vi "set_material_parameters_cluster.vi"(8 "error in (no error)":errorcluster, 9 "Material parameters":T1, 10 "Material number":u8, 11 "VISA resource name":refnum<visa-resource-name>) -> (0 "error out":errorcluster, 3 "VISA resource name out":refnum<visa-resource-name>)   [LabVIEW 2018]
doc: "Set the density of a material."
uses:
  Low Level/material_parameter_ring.ctl
  Low Level/material_parameters.ctl
panel:
  out "Label.Text":string
  in  "Material parameter":T2 items=["Density (g/cc)", "Z-Ratio", "Master Tooling (%)", "Control Loop", "Process Gain (A/s/%)", "Time Constant (s)", "Dead Time (s)", "Source", "Maximum Power (%)", "Minimum Power (%)", "Max Power Option", "PreCond Soak Power (%)", "PreCond Rise Time (s) (mm:ss)", "PreCond Soak Time (s) (mm:ss)", "Soak Power 1 (%)", "Rise Time 1 (s) (mm:ss)", "Soak Time 1 (s) (mm:ss)", "Soak Power 2 (%)", "Rise Time 2 (s) (mm:ss)", "Soak Time 2 (s) (mm:ss)", "Auto Soak 2", "Dep After Pre-Dep", "Delay Option", "Control Delay Time (s) (mm:ss)", "Shutter Delay Accur (%)", "Transfer Sensor", "Transfer Tooling (%)", "Feed Power (%)", "Feed Ramp Time (s) (mm:ss)", "Feed Time (s) (mm:ss)", "Idle Power (%)", "Idle Ramp Time (s) (mm:ss)", "Rate (A/s)", "Time Limit (s) (mm:ss)", "Rate Filter Time (s)", "Time Power Avg Time (minutes)", "Ion Assist Deposit", "On Final Thickness", "Ramp 1 Rate (A/s)", "Start Ramp 1 (kA)", "Ramp 1 Time (s) (mm:ss)", "Ramp 2 Rate (A/s)", "Start Ramp 2 (kA)", "Ramp 2 Time (s) (mm:ss)", "RateWatcher Option", "RateWatcher Time (s) (mm:ss)", "RateWatcher Accuracy (%)", "Multipoint", "Aggregate Multiplier", "Sensor 1 Failure Action", "Sensor 2 Failure Action", "Sensor 3 Failure Action", "Sensor 4 Failure Action", "Sensor 5 Failure Action", "Sensor 6 Failure Action", "Sensor 7 Failure Action", "Sensor 8 Failure Action", "Sensor 1 Failure Trigger", "Sensor 2 Failure Trigger", "Sensor 3 Failure Trigger", "Sensor 4 Failure Trigger", "Sensor 5 Failure Trigger", "Sensor 6 Failure Trigger", "Sensor 7 Failure Trigger", "Sensor 8 Failure Trigger", "Sensor 1 Weight (%)", "Sensor 2 Weight (%)", "Sensor 3 Weight (%)", "Sensor 4 Weight (%)", "Sensor 5 Weight (%)", "Sensor 6 Weight (%)", "Sensor 7 Weight (%)", "Sensor 8 Weight (%)", "Sensor 1 Tooling (%)", "Sensor 2 Tooling (%)", "Sensor 3 Tooling (%)", "Sensor 4 Tooling (%)", "Sensor 5 Tooling (%)", "Sensor 6 Tooling (%)", "Sensor 7 Tooling (%)", "Sensor 8 Tooling (%)", "Sensor 1 CrystalTwo Tooling (%)", "Sensor 2 CrystalTwo Tooling (%)", "Sensor 3 CrystalTwo Tooling (%)", "Sensor 4 CrystalTwo Tooling (%)", "Sensor 5 CrystalTwo Tooling (%)", "Sensor 6 CrystalTwo Tooling (%)", "Sensor 7 CrystalTwo Tooling (%)", "Sensor 8 CrystalTwo Tooling (%)", "Sensor 1 Cal Thickness (kA)", "Sensor 2 Cal Thickness (kA)", "Sensor 3 Cal Thickness (kA)", "Sensor 4 Cal Thickness (kA)", "Sensor 5 Cal Thickness (kA)", "Sensor 6 Cal Thickness (kA)", "Sensor 7 Cal Thickness (kA)", "Sensor 8 Cal Thickness (kA)", "Sensor 1 Xtal Position First", "Sensor 2 Xtal Position First", "Sensor 3 Xtal Position First", "Sensor 4 Xtal Position First", "Sensor 5 Xtal Position First", "Sensor 6 Xtal Position First", "Sensor 7 Xtal Position First", "Sensor 8 Xtal Position First", "Sensor 1 Xtal Position Last", "Sensor 2 Xtal Position Last", "Sensor 3 Xtal Position Last", "Sensor 4 Xtal Position Last", "Sensor 5 Xtal Position Last", "Sensor 6 Xtal Position Last", "Sensor 7 Xtal Position Last", "Sensor 8 Xtal Position Last", "Sensor", "Failure Action", "CrystalTwo Tooling (%)", "Xtal Position First", "Xtal Position Last", "Backup Sensor", "Backup Tooling (%)", "Quality Percent (%)", "Quality Counts", "Stability Single (Hz)", "Stability Total (Hz)", "Recorder Output", "Recorder Function", "Recorder Range"]
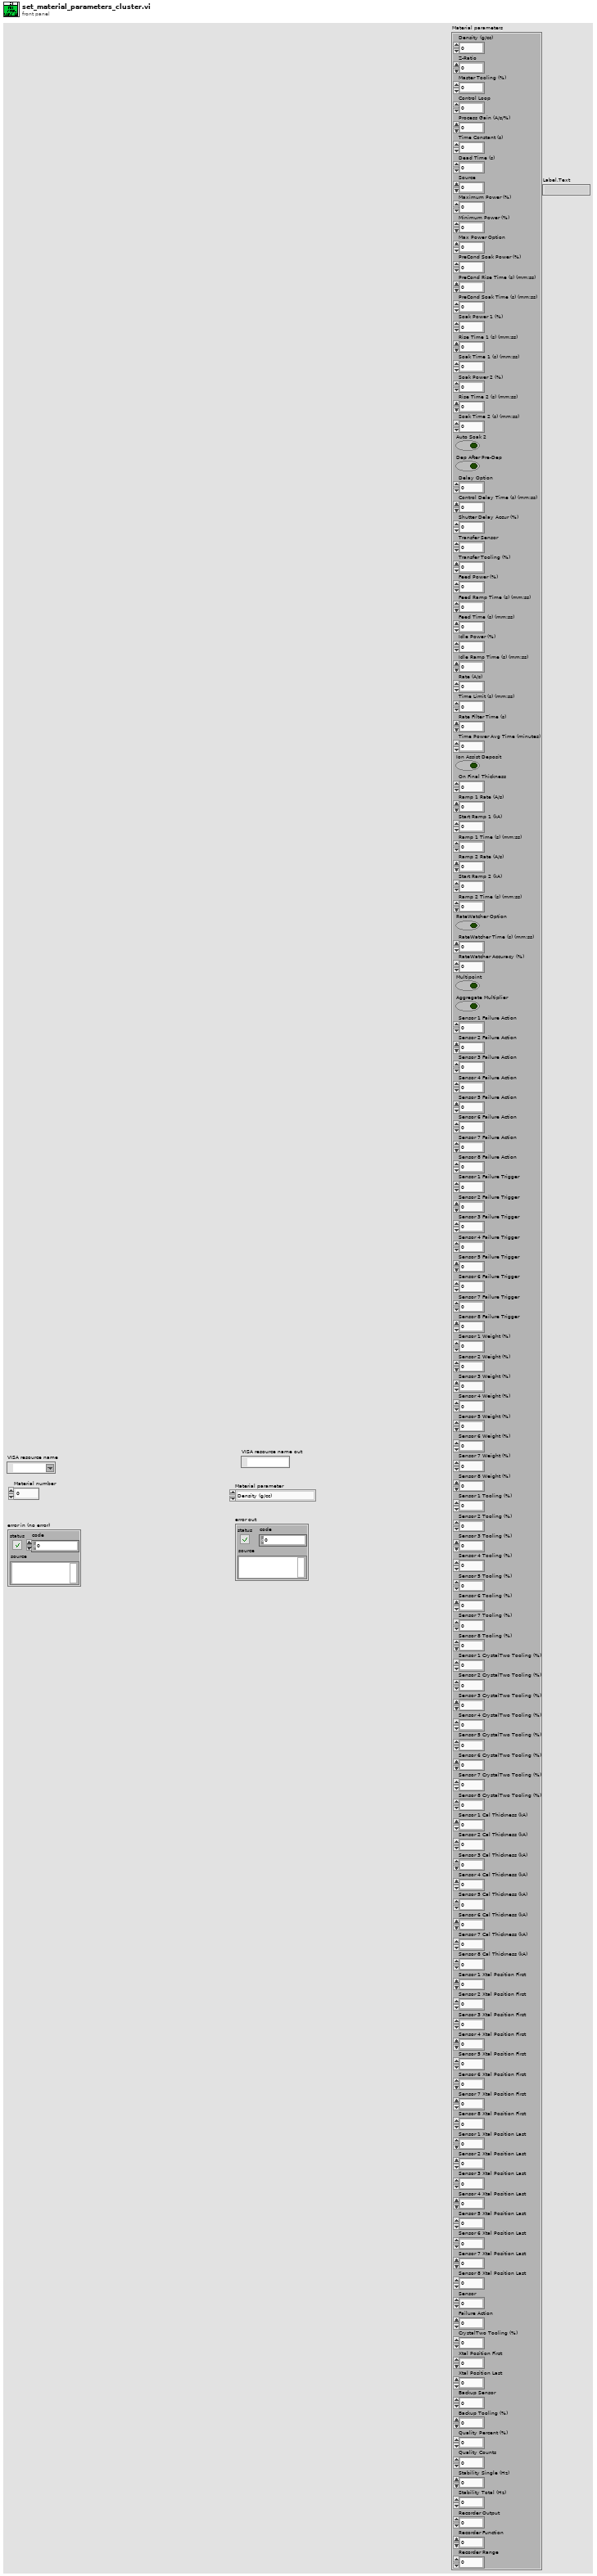
[diagram p1: front panel]
types:
  T1 = typedef "material_parameters.ctl" = cluster{"Density (g/cc)":sgl, "Z-Ratio":sgl, "Master Tooling (%)":sgl, "Control Loop":u8, "Process Gain (A/s/%)":sgl, "Time Constant (s)":sgl, "Dead Time (s)":sgl, "Source":u8, "Maximum Power (%)":sgl, "Minimum Power (%)":sgl, "Max Power Option":u8, "PreCond Soak Power (%)":sgl, "PreCond Rise Time (s) (mm:ss)":u16, "PreCond Soak Time (s) (mm:ss)":u16, "Soak Power 1 (%)":sgl, "Rise Time 1 (s) (mm:ss)":u16, "Soak Time 1 (s) (mm:ss)":u16, "Soak Power 2 (%)":sgl, "Rise Time 2 (s) (mm:ss)":u16, "Soak Time 2 (s) (mm:ss)":u16, "Auto Soak 2":bool, "Dep After Pre-Dep":bool, "Delay Option":u8, "Control Delay Time (s) (mm:ss)":u16, "Shutter Delay Accur (%)":u8, "Transfer Sensor":u8, "Transfer Tooling (%)":sgl, "Feed Power (%)":sgl, "Feed Ramp Time (s) (mm:ss)":u16, "Feed Time (s) (mm:ss)":u16, "Idle Power (%)":sgl, "Idle Ramp Time (s) (mm:ss)":u16, "Rate (A/s)":sgl, "Time Limit (s) (mm:ss)":u16, "Rate Filter Time (s)":u8, "Time Power Avg Time (minutes)":u8, "Ion Assist Deposit":bool, "On Final Thickness":u8, "Ramp 1 Rate (A/s)":sgl, "Start Ramp 1 (kA)":sgl, "Ramp 1 Time (s) (mm:ss)":u16, "Ramp 2 Rate (A/s)":sgl, "Start Ramp 2 (kA)":sgl, "Ramp 2 Time (s) (mm:ss)":u16, "RateWatcher Option":bool, "RateWatcher Time (s) (mm:ss)":u16, "RateWatcher Accuracy (%)":u8, "Multipoint":bool, "Aggregate Multiplier":bool, "Sensor 1 Failure Action":u8, "Sensor 2 Failure Action":u8, "Sensor 3 Failure Action":u8, "Sensor 4 Failure Action":u8, "Sensor 5 Failure Action":u8, "Sensor 6 Failure Action":u8, "Sensor 7 Failure Action":u8, "Sensor 8 Failure Action":u8, "Sensor 1 Failure Trigger":u8, "Sensor 2 Failure Trigger":u8, "Sensor 3 Failure Trigger":u8, "Sensor 4 Failure Trigger":u8, "Sensor 5 Failure Trigger":u8, "Sensor 6 Failure Trigger":u8, "Sensor 7 Failure Trigger":u8, "Sensor 8 Failure Trigger":u8, "Sensor 1 Weight (%)":sgl, "Sensor 2 Weight (%)":sgl, "Sensor 3 Weight (%)":sgl, "Sensor 4 Weight (%)":sgl, "Sensor 5 Weight (%)":sgl, "Sensor 6 Weight (%)":sgl, "Sensor 7 Weight (%)":sgl, "Sensor 8 Weight (%)":sgl, "Sensor 1 Tooling (%)":sgl, "Sensor 2 Tooling (%)":sgl, "Sensor 3 Tooling (%)":sgl, "Sensor 4 Tooling (%)":sgl, "Sensor 5 Tooling (%)":sgl, "Sensor 6 Tooling (%)":sgl, "Sensor 7 Tooling (%)":sgl, "Sensor 8 Tooling (%)":sgl, "Sensor 1 CrystalTwo Tooling (%)":sgl, "Sensor 2 CrystalTwo Tooling (%)":sgl, "Sensor 3 CrystalTwo Tooling (%)":sgl, "Sensor 4 CrystalTwo Tooling (%)":sgl, "Sensor 5 CrystalTwo Tooling (%)":sgl, "Sensor 6 CrystalTwo Tooling (%)":sgl, "Sensor 7 CrystalTwo Tooling (%)":sgl, "Sensor 8 CrystalTwo Tooling (%)":sgl, "Sensor 1 Cal Thickness (kA)":sgl, "Sensor 2 Cal Thickness (kA)":sgl, "Sensor 3 Cal Thickness (kA)":sgl, "Sensor 4 Cal Thickness (kA)":sgl, "Sensor 5 Cal Thickness (kA)":sgl, "Sensor 6 Cal Thickness (kA)":sgl, "Sensor 7 Cal Thickness (kA)":sgl, "Sensor 8 Cal Thickness (kA)":sgl, "Sensor 1 Xtal Position First":u8, "Sensor 2 Xtal Position First":u8, "Sensor 3 Xtal Position First":u8, "Sensor 4 Xtal Position First":u8, "Sensor 5 Xtal Position First":u8, "Sensor 6 Xtal Position First":u8, "Sensor 7 Xtal Position First":u8, "Sensor 8 Xtal Position First":u8, "Sensor 1 Xtal Position Last":u8, "Sensor 2 Xtal Position Last":u8, "Sensor 3 Xtal Position Last":u8, "Sensor 4 Xtal Position Last":u8, "Sensor 5 Xtal Position Last":u8, "Sensor 6 Xtal Position Last":u8, "Sensor 7 Xtal Position Last":u8, "Sensor 8 Xtal Position Last":u8, "Sensor":u8, "Failure Action":u8, "CrystalTwo Tooling (%)":sgl, "Xtal Position First":u8, "Xtal Position Last":u8, "Backup Sensor":u8, "Backup Tooling (%)":sgl, "Quality Percent (%)":u8, "Quality Counts":u8, "Stability Single (Hz)":u8, "Stability Total (Hz)":u8, "Recorder Output":u8, "Recorder Function":u8, "Recorder Range":u8}
  T2 = typedef "material_parameter_ring.ctl" = u16
  T3 = typedef "LVStringsAndValuesArrayTypeDef_U16.ctl" = cluster{"String":string, "Value":u16}[]
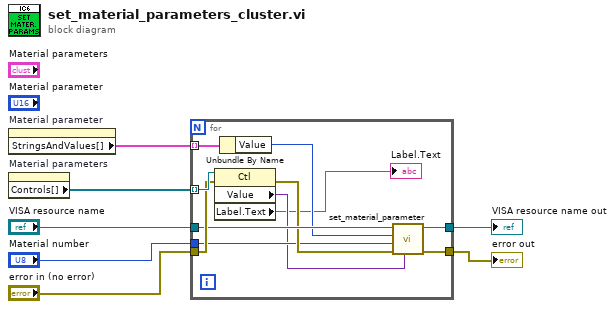
[diagram p0: block diagram]
diagram:
  n1 = property on="Material parameter" class="Ring (strict)"() -> ("StringsAndValues[]"=w4:T3)  [unwired: 2 in, 2 out]
  n2 = property on="Material parameters" class="Clust (strict)"() -> ("Controls[]"=w3:refnum<vi>[])  [unwired: 2 in, 2 out]
  n3 = for {
    tunnel: "VISA resource name" -> [w15]
    tunnel: [w10] -> w6
    tunnel: [w9] -> w1
    tunnel: "error in (no error)" -> [w17]
    tunnel: "Material number" -> [w12]
    tunnel: w4 -> [w16] mode=indexing
    tunnel: w3 -> [w18] mode=indexing
    n4 = property class="Ctl"(reference=w18, error in=w17) -> (error out=w14:errorcluster, "Value"=w11:variant, "Label.Text"=→"Label.Text":string)  [unwired: 1 out]
    n5 = Unbundle By Name(w16) -> ("Value"=w13:u16)
    n6 = call "set_material_parameter.vi"("Parameter value"=w11, "error in (no error)"=w14, "Material number"=w12, "Material parameter"=w13, "VISA resource name"=w15) -> ("error out"=w9:errorcluster, "VISA resource name out"=w10:refnum<visa-resource-name>)  [unwired: 5 in]
  }
  "error out" <- w1
  "VISA resource name out" <- w6
